vi "MultiPeak Lorentzian fit.vi"(0 "Data":cluster{dbl[], dbl[]}(graph)={[-8.499999999999992e-05, -7.999999999999991e-05, -7.500000000000001e-05, -7e-05, -6.499999999999998e-05, -5.999999999999996e-05, -5.499999999999995e-05, -4.9999999999999935e-05, -4.499999999999992e-05, -3.999999999999991e-05, -3.4999999999999895e-05, -2.999999999999999e-05, -2.4999999999999977e-05, -1.9999999999999964e-05, -1.4999999999999951e-05, -9.999999999999938e-06, -4.999999999999925e-06, 8.809142651444724e-20, 5.000000000000101e-06, 1.0000000000000114e-05, 1.5000000000000019e-05, 2.0000000000000032e-05, 2.5000000000000045e-05, 3.0000000000000167e-05, 3.499999999999996e-05, 3.9999999999999976e-05, 4.499999999999999e-05, 5e-05, 5.5000000000000016e-05, 6.000000000000003e-05, 6.500000000000003e-05, 7.000000000000005e-05, 7.500000000000006e-05, 8.000000000000007e-05, 8.500000000000009e-05, 9.00000000000001e-05, 9.500000000000011e-05, 0.00010000000000000013, 0.00010500000000000014, 0.00011000000000000015, 0.00011500000000000017, 0.00011999999999999996, 0.00012499999999999998, 0.00013, 0.000135, 0.00014000000000000001, 0.00014500000000000003, 0.00015000000000000004, 0.00015500000000000005, 0.00016000000000000007, 0.00016500000000000008, 0.0001700000000000001, 0.0001750000000000001, 0.00018000000000000012, 0.00018500000000000013, 0.00019000000000000015, 0.00019500000000000016, 0.00020000000000000017, 0.00020499999999999997, 0.00020999999999999998, 0.000215], [0.0012150575654108651, 0.001198658781387788, 0.0011426384093853204, 0.0010813452811549607, 0.0010303635282890781, 0.0009901242148328533, 0.0009655793533614787, 0.0009637788368138997, 0.0010005358746802097, 0.0010629165364520092, 0.0011453292663476753, 0.0012282965012078144, 0.0013016140805626642, 0.0013824481174704287, 0.0014643235971013074, 0.001551428490294265, 0.0016410212376952622, 0.0017011308416755618, 0.0017405751692456835, 0.0017894187526559019, 0.0018475004228560138, 0.001935889200879927, 0.0020558944722601385, 0.0022018521313563566, 0.0023273539722724924, 0.0024094326874369767, 0.0024636017852976066, 0.002504959490390853, 0.002523953570272467, 0.0025357303860099067, 0.002533784895930486, 0.002531304880465543, 0.002510967573955287, 0.0024732435245279774, 0.002443623217043697, 0.0023599211252369095, 0.0022706549323664466, 0.002214470491667274, 0.002125513838829537, 0.00201932637179927, 0.0019171339548864448, 0.0018332672503242942, 0.0017464983694980517, 0.0016410088936650942, 0.0015556613369979762, 0.0014804206312365406, 0.0014134274487672173, 0.001353115324136875, 0.001296938061612269, 0.0012362798726307397, 0.0011647776947571107, 0.0011200248904945148, 0.001093147276680698, 0.0010656806623489281, 0.0010521925231414086, 0.0010354102047782196, 0.0010134722469805815, 0.0009927942501985478, 0.0009831918813237074, 0.000993569602746048, 0.0010334011217177546]}, 1 "Enable peak doubling":bool=TRUE, 2 "range":T1={"x1"=-0.6878048780487804, "y1"=-55263.15789473684, "x 2"=0.47317073170731705, "y 2"=53947.36842105264}, 5 "Formula":string="a+4*b/(exp(1.7628*(x-c)/d)+exp(-1.7628*(x-c)/d))^2 ", 7 "Field (Oe)":dbl=39767.44186046513, 9 "model and initial parameter input\nuse \"XXX\" if void":T3={"a (constant)"="a", "b (amplitude)"="b", "c (position)"="c", "d (width)"="d", "ai"=0.0, "bi"=0.0, "ci"=0.0, "di"=0.002} {"di" format="%.3f"; "ci" format="%.3f"; "bi" format="%.3p"; "ai" format="%.2p"}, 11 "PD threshold":dbl format="%.2p", 12 "PD width":i32=10 min=3) -> (4 "Fit":cluster{dbl[], "best nonlinear fit":dbl[]}[](graph)=[{[-8.499999999999992e-05, -7.999999999999991e-05, -7.500000000000001e-05, -7e-05, -6.499999999999998e-05, -5.999999999999996e-05, -5.499999999999995e-05, -4.9999999999999935e-05, -4.499999999999992e-05, -3.999999999999991e-05, -3.4999999999999895e-05, -2.999999999999999e-05, -2.4999999999999977e-05, -1.9999999999999964e-05, -1.4999999999999951e-05, -9.999999999999938e-06, -4.999999999999925e-06, 8.809142651444724e-20, 5.000000000000101e-06, 1.0000000000000114e-05, 1.5000000000000019e-05, 2.0000000000000032e-05, 2.5000000000000045e-05, 3.0000000000000167e-05, 3.499999999999996e-05, 3.9999999999999976e-05, 4.499999999999999e-05, 5e-05, 5.5000000000000016e-05, 6.000000000000003e-05, 6.500000000000003e-05, 7.000000000000005e-05, 7.500000000000006e-05, 8.000000000000007e-05, 8.500000000000009e-05, 9.00000000000001e-05, 9.500000000000011e-05, 0.00010000000000000013, 0.00010500000000000014, 0.00011000000000000015, 0.00011500000000000017, 0.00011999999999999996, 0.00012499999999999998, 0.00013, 0.000135, 0.00014000000000000001, 0.00014500000000000003, 0.00015000000000000004, 0.00015500000000000005, 0.00016000000000000007, 0.00016500000000000008, 0.0001700000000000001, 0.0001750000000000001, 0.00018000000000000012, 0.00018500000000000013, 0.00019000000000000015, 0.00019500000000000016, 0.00020000000000000017, 0.00020499999999999997, 0.00020999999999999998, 0.000215], "best nonlinear fit"=[0.0009718951839726664, 0.0009807254858543823, 0.0009616076605343897, 0.0009333705018249478, 0.0009129931681906823, 0.000909763379760772, 0.0009260752896536717, 0.0009606338293882525, 0.0010110188438919138, 0.00107496449821926, 0.0011507542027808617, 0.0012371991520140234, 0.0013334777164069607, 0.0014389569248984503, 0.0015530359178241016, 0.0016750182813155834, 0.0018040103672834111, 0.0019388420707677372, 0.00207800877224406, 0.0022196357214930174, 0.002361468065228045, 0.0025008905889973045, 0.0026349808385329318, 0.002760597510997979, 0.0028745029297172096, 0.0029735143382420446, 0.003054674246520122, 0.003115425949217566, 0.00315377753993939, 0.0031684370891274863, 0.0031589036174095096, 0.003125503025407498, 0.0030693645891025556, 0.0029923408761758996, 0.0028968806583283737, 0.0027858693960421755, 0.002662454390667553, 0.0025298715492623517, 0.0023912882630169243, 0.002249672921582608, 0.0021076969825550677, 0.0019676711178937966, 0.001831513364386468, 0.0017007447194402514, 0.001576506285790725, 0.001459591726268164, 0.0013504891872005128, 0.0012494277072594559, 0.0011564241990958423, 0.0010713281841576634, 0.0009938624521659315, 0.0009236586396038637, 0.0008602873545952086, 0.0008032829267293593, 0.0007521631544091965, 0.0007064445906497542, 0.0006656539827412946, 0.0006293364901872711, 0.0005970612721299563, 0.000568424977978641, 0.0005430536061055539]}, {[-8.499999999999992e-05, -7.999999999999991e-05, -7.500000000000001e-05, -7e-05, -6.499999999999998e-05, -5.999999999999996e-05, -5.499999999999995e-05, -4.9999999999999935e-05, -4.499999999999992e-05, -3.999999999999991e-05, -3.4999999999999895e-05, -2.999999999999999e-05, -2.4999999999999977e-05, -1.9999999999999964e-05, -1.4999999999999951e-05, -9.999999999999938e-06, -4.999999999999925e-06, 8.809142651444724e-20, 5.000000000000101e-06, 1.0000000000000114e-05, 1.5000000000000019e-05, 2.0000000000000032e-05, 2.5000000000000045e-05, 3.0000000000000167e-05, 3.499999999999996e-05, 3.9999999999999976e-05, 4.499999999999999e-05, 5e-05, 5.5000000000000016e-05, 6.000000000000003e-05, 6.500000000000003e-05, 7.000000000000005e-05, 7.500000000000006e-05, 8.000000000000007e-05, 8.500000000000009e-05, 9.00000000000001e-05, 9.500000000000011e-05, 0.00010000000000000013, 0.00010500000000000014, 0.00011000000000000015, 0.00011500000000000017, 0.00011999999999999996, 0.00012499999999999998, 0.00013, 0.000135, 0.00014000000000000001, 0.00014500000000000003, 0.00015000000000000004, 0.00015500000000000005, 0.00016000000000000007, 0.00016500000000000008, 0.0001700000000000001, 0.0001750000000000001, 0.00018000000000000012, 0.00018500000000000013, 0.00019000000000000015, 0.00019500000000000016, 0.00020000000000000017, 0.00020499999999999997, 0.00020999999999999998, 0.000215], "best nonlinear fit"=[0.000989689814848765, 0.0009691184141790208, 0.0009366814384494319, 0.0009211036423827158, 0.0009263722031401187, 0.0009445966388776419, 0.0009696289439432098, 0.000992032437226056, 0.0010164205448619874, 0.001046657083728515, 0.0010862347078188814, 0.0011332970048991335, 0.0011997862974852938, 0.0012949918371966656, 0.001418474742517191, 0.0015812404841218492, 0.0017676702020836762, 0.001961275405311842, 0.002171201133245579, 0.0023792297464750147, 0.0025461522166526284, 0.002674004984876295, 0.0027969468914240854, 0.0029046334176933536, 0.0029750408059281484, 0.003019636865052686, 0.0030181976868652077, 0.002970402911603623, 0.0028998850653752556, 0.0028692674041395257, 0.002887874691658434, 0.0029727149791749707, 0.0030509519871012077, 0.003078767698694361, 0.00305866218326655, 0.002964500307352822, 0.0028210241662788584, 0.0026652309117736156, 0.0025033186072926125, 0.0023465893570533388, 0.002176728611772454, 0.001991535600650964, 0.0018155595228638325, 0.0016408583384044829, 0.0014856986821473453, 0.0013489469222139202, 0.0012394448202315484, 0.0011564229466427634, 0.0010753411266288153, 0.0010053852995606425, 0.0009444950046100983, 0.0008825159005678181, 0.0008246355886464278, 0.0007782164102647071, 0.0007506957685204472, 0.000728846188097151, 0.0007052979668229569, 0.000689497674504493, 0.0006869125707686534, 0.0006897761061261346, 0.0007007193940464603]}], 6 "best fit parameters":dbl[](array[numeric])=[0.00017751423776879837, 0.00038127860723276904, -8.528154856218626e-05, 3.738209460996479e-05, 0.0028135439197028837, 6.053132635732174e-05, 0.00013421483148268372], 8 "PD peak position":dbl[](array[numeric])=[-4.999999999999925e-06, 6.000000000000003e-05], 10 "# of peaks":i32=2, 14 "R-square":dbl=0.9832767875868196, 15 "std deviation":dbl[](array[numeric])=[3.738389415758166e-05, 0.00012746351087395422, 1.538590755264726e-05, 2.4846960511995104e-05, 7.093705091399118e-05, 8.710626646709724e-07, 4.935700356045006e-06])   [LabVIEW 2016]
uses:
  <vilib>/Analysis/Matrix/Datatypes/RealMatrix.ctl
  <vilib>/gmath/NumericalOptimization/Nonlinear Curve Fit LM formula string.vi
  <vilib>/gmath/NI_Gmath.lvlib
  <vilib>/Analysis/NI_AAL_SigProc.lvlib
  <vilib>/Analysis/Matrix/NI_Matrix.lvlib
panel:
  out "residue":cluster{dbl[], dbl[]}(graph)={[-8.499999999999992e-05, -7.999999999999991e-05, -7.500000000000001e-05, -7e-05, -6.499999999999998e-05, -5.999999999999996e-05, -5.499999999999995e-05, -4.9999999999999935e-05, -4.499999999999992e-05, -3.999999999999991e-05, -3.4999999999999895e-05, -2.999999999999999e-05, -2.4999999999999977e-05, -1.9999999999999964e-05, -1.4999999999999951e-05, -9.999999999999938e-06, -4.999999999999925e-06, 8.809142651444724e-20, 5.000000000000101e-06, 1.0000000000000114e-05, 1.5000000000000019e-05, 2.0000000000000032e-05, 2.5000000000000045e-05, 3.0000000000000167e-05, 3.499999999999996e-05, 3.9999999999999976e-05, 4.499999999999999e-05, 5e-05, 5.5000000000000016e-05, 6.000000000000003e-05, 6.500000000000003e-05, 7.000000000000005e-05, 7.500000000000006e-05, 8.000000000000007e-05, 8.500000000000009e-05, 9.00000000000001e-05, 9.500000000000011e-05, 0.00010000000000000013, 0.00010500000000000014, 0.00011000000000000015, 0.00011500000000000017, 0.00011999999999999996, 0.00012499999999999998, 0.00013, 0.000135, 0.00014000000000000001, 0.00014500000000000003, 0.00015000000000000004, 0.00015500000000000005, 0.00016000000000000007, 0.00016500000000000008, 0.0001700000000000001, 0.0001750000000000001, 0.00018000000000000012, 0.00018500000000000013, 0.00019000000000000015, 0.00019500000000000016, 0.00020000000000000017, 0.00020499999999999997, 0.00020999999999999998, 0.000215], [1.7794630876098662e-05, -1.1607071675361568e-05, -2.492622208495783e-05, -1.2266859442232043e-05, 1.337903494943646e-05, 3.4833259116869844e-05, 4.3553654289538125e-05, 3.13986078378035e-05, 5.401700970073583e-06, -2.830741449074488e-05, -6.451949496198033e-05, -0.00010390214711488983, -0.0001336914189216669, -0.00014396508770178466, -0.00013456117530691054, -9.377779719373417e-05, -3.634016519973491e-05, 2.2433334544104747e-05, 9.31923610015188e-05, 0.00015959402498199726, 0.00018468415142458344, 0.00017311439587899043, 0.00016196605289115363, 0.00014403590669537485, 0.00010053787621093881, 4.6122526810641554e-05, -3.647655965491412e-05, -0.00014502303761394298, -0.00025389247456413444, -0.0002991696849879606, -0.0002710289257510756, -0.0001527880462325274, -1.8412602001347846e-05, 8.642682251846145e-05, 0.00016178152493817642, 0.00017863091131064667, 0.00015856977561130555, 0.0001353593625112639, 0.0001120303442756882, 9.691643547073093e-05, 6.903162921738631e-05, 2.3864482757167318e-05, -1.5953841522635404e-05, -5.988638103576857e-05, -9.080760364337968e-05, -0.00011064480405424378, -0.00011104436696896436, -9.30047606166925e-05, -8.108307246702698e-05, -6.594288459702089e-05, -4.9367447555833245e-05, -4.1142739036045665e-05, -3.565176594878079e-05, -2.5066516464652207e-05, -1.4673858887493448e-06, 2.2401597447396803e-05, 3.964398408166231e-05, 6.016118431722195e-05, 8.985129863869705e-05, 0.0001213511281474936, 0.0001576657879409064]}
  out "covariance":T2=[[0.09601636295019793, -0.11196924282221532, 0.0019290808585169803, -0.008016159684207873, -0.15830836798965434, -0.0003679452768878755, -0.01111098483349951], [-0.11196924282221542, 1.1162151876482052, -0.09483397785102357, 0.10825444863719698, 0.20981268047054838, 0.0013201880795881457, 0.009063931764684398], [0.001929080858517002, -0.09483397785102358, 0.01626381447167083, -0.023123770063261814, -0.005876578599017109, -0.00015274264582045002, 0.000286765518797958], [-0.008016159684207928, 0.10825444863719715, -0.023123770063261818, 0.042415316674133494, 0.02100058943438996, 0.0003972550480277107, -0.00044102254426060404], [-0.15830836798965442, 0.20981268047054832, -0.005876578599017081, 0.021000589434389854, 0.34571835125452366, 0.0007469589653986517, 0.014676057612944117], [-0.0003679452768878726, 0.0013201880795881745, -0.00015274264582044948, 0.00039725504802770573, 0.0007469589653986541, 5.212846938596066e-05, 2.0363029410124748e-05], [-0.0111109848334995, 0.009063931764684367, 0.0002867655187979612, -0.00044102254426061195, 0.014676057612944087, 2.0363029410124728e-05, 0.0016736850862781277]] format="%#_5g"
  out "Initial parameters":dbl[](array[numeric])=[0.0, 0.0016410212376952622, -4.999999999999925e-06, 0.002, 0.0025357303860099067, 6.000000000000003e-05, 0.002]
  out "PD Amplitudes":dbl[](array[numeric])=[0.0016410212376952622, 0.0025357303860099067]
  in  "model description output":T4={"model"="a+4*b0/(exp(1.7628*(x-c0)/d0)+exp(-1.7628*(x-c0)/d0))^2 +a+4*b1/(exp(1.7628*(x-c1)/d1)+exp(-1.7628*(x-c1)/d1))^2 ", "Parameters"=["a", "b0", "c0", "d0", "b1", "c1", "d1"], "x"="x"}
  # "This program can fit any peak function as far as the number of parameters<=4\nuse \"XXX\" and \"NaN\" if the corresponding parameter is not in use.\n\n4 parameter functions:\nLorentzian: a+b*d^2/(4*x^2-8*c*x+4*c^2+d^2)\n\nHyperbolic cosine: a+4*b/(exp(1.7628*(x-c)/d)+exp(-1.7628*(x-c)/d))^2"
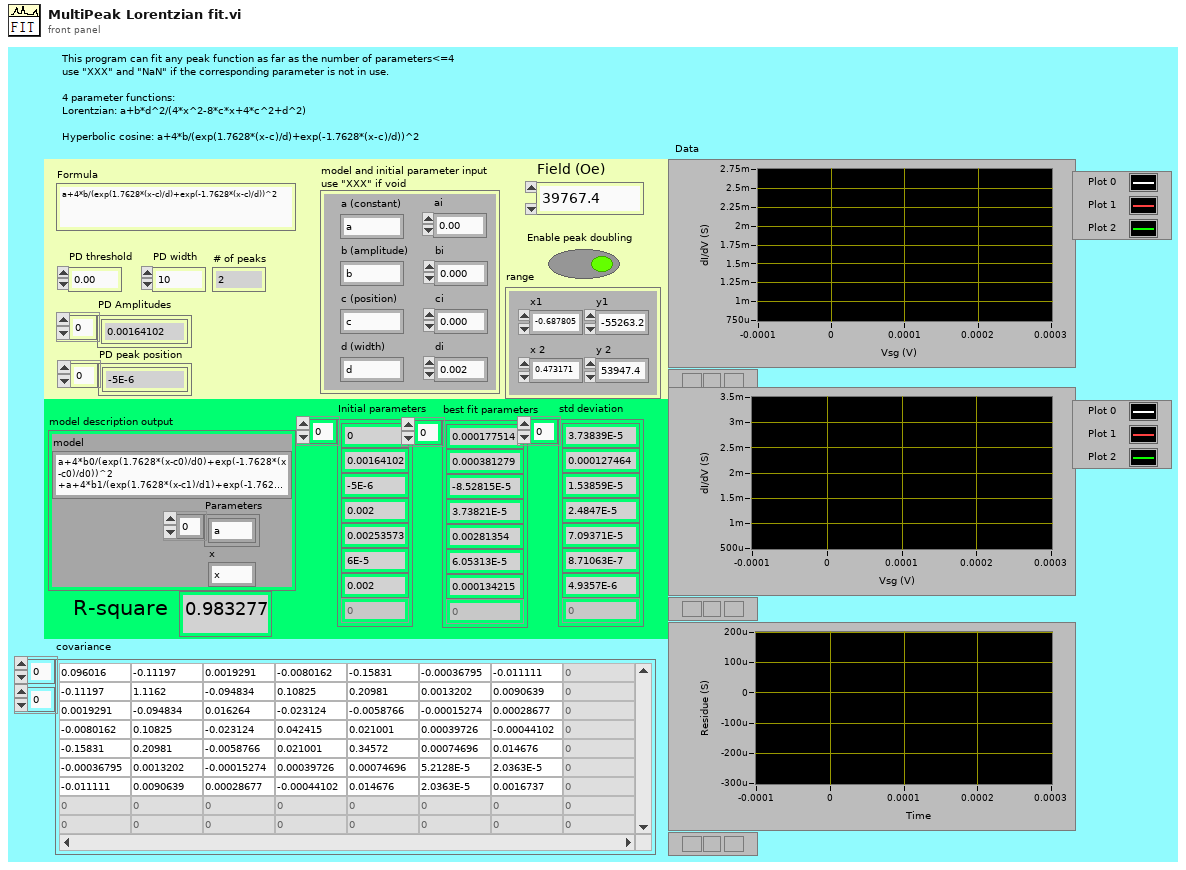
[diagram p1: front panel]
types:
  T1 = cluster{"x1":dbl, "y1":dbl, "x 2":dbl, "y 2":dbl}
  T2 = typedef "NI_Matrix.lvlib/RealMatrix.ctl" = dbl[][]
  T3 = cluster{"a (constant)":string, "b (amplitude)":string, "c (position)":string, "d (width)":string, "ai":dbl, "bi":dbl, "ci":dbl, "di":dbl}
  T4 = cluster{"model":string, "Parameters":string[], "x":string}
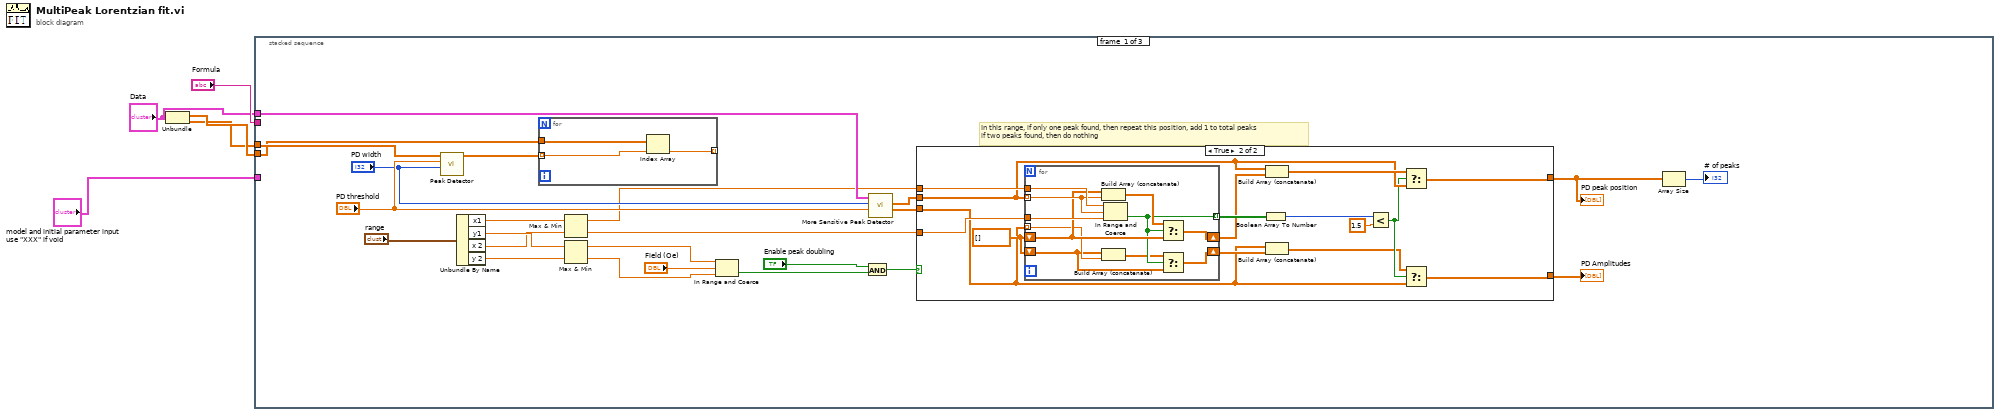
[diagram p0: block diagram]
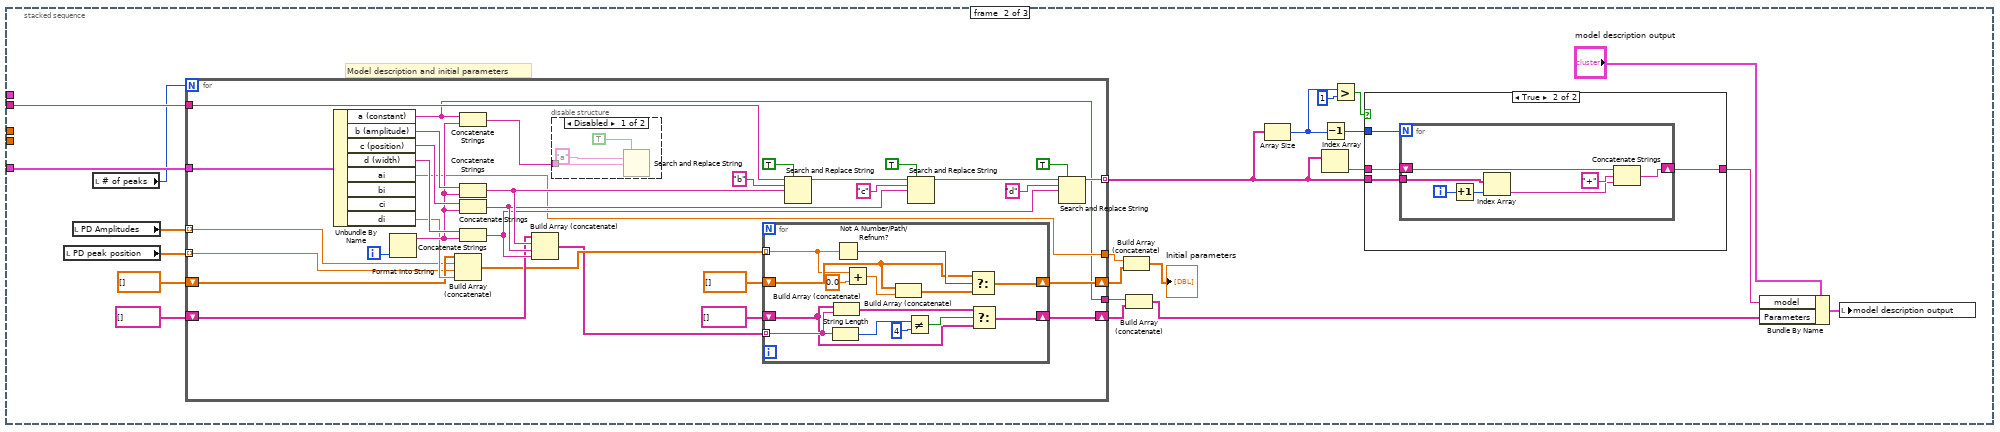
[diagram p3: hidden frame]
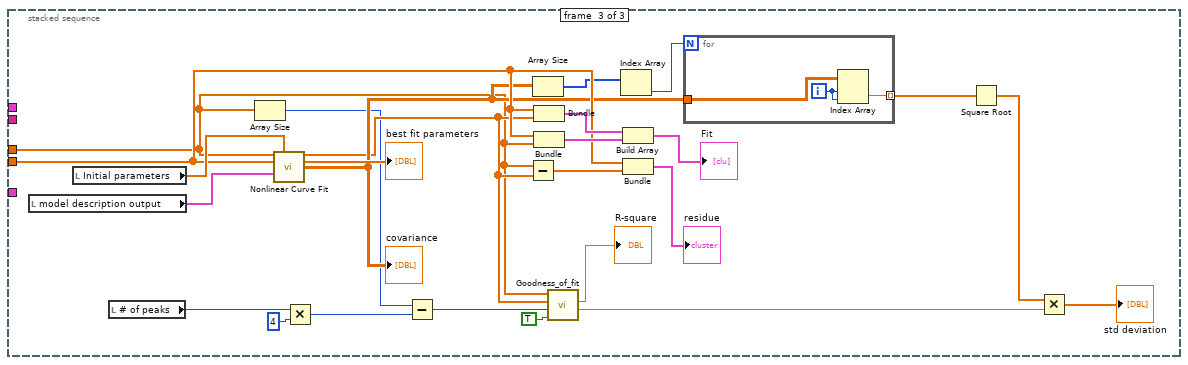
[diagram p6: hidden frame]
diagram:
  n1 = Unbundle("Data") -> (w3:dbl[], w1:dbl[])
  n2 = stacked-sequence {
    tunnel: "Formula" -> [_ w82 _]
    tunnel: "model and initial parameter input\nuse \"XXX\" if void" -> [_ w81 _]
    tunnel: w3 -> [w27 _ w162]
    tunnel: w1 -> [w29 _ w154]
    tunnel: "Data" -> [w25 _ _]
    frame #0 {
      # "In this range, if only one peak found, then repeat this position, add 1 to total peaks\nif two peaks found, then do nothing"
      n3 = call <vilib>:"Peak Detector.vi"("width"="PD width", "threshold"="PD threshold", "X"=w29) -> ("Locations"=w26:dbl[])  [unwired: 4 in, 4 out]
      n4 = Unbundle By Name("range") -> ("x1"=w9:dbl, "y1"=w16:dbl, "x 2"=w8:dbl, "y 2"=w15:dbl)
      n5 = for {
        tunnel: w27 -> [w60]
        tunnel: w26 -> [w59] mode=indexing
        tunnel: [w58] -> _ mode=indexing
        n6 = Index Array(array=w60, index=w59) -> (element=w58:dbl)
      }
      n7 = Max & Min(x=w9, y=w8) -> (max(x,y)=w7:dbl, min(x,y)=w6:dbl)
      n8 = Max & Min(x=w16, y=w15) -> (max(x,y)=w14:dbl, min(x,y)=w13:dbl)
      n9 = In Range and Coerce(upper limit=w14, x="Field (Oe)", lower limit=w13) -> (In Range?=w11:bool)  [unwired: 1 out]
      n10 = And(x="Enable peak doubling", y=w11) -> (x .and. y?=w10:bool)
      n11 = call "More Sensitive Peak Detector.vi"("PD threshold"="PD threshold", "Smooth points"="PD width", "Input XY"=w25) -> ("Amplitudes"=w19:dbl[], "Positions"=w21:dbl[])  [unwired: 6 in, 1 out]
      n12 = case shown="True" w10 {
        tunnel: w21 -> [w31 w37]
        tunnel: [w31 w36] -> w20
        tunnel: w19 -> [w30 w32]
        tunnel: [w30 w33] -> w18
        tunnel: w7 -> [_ w46]
        tunnel: w6 -> [_ w45]
        frame False {
        }
        frame True {
          w40 = dbl[] []
          n13 = for {
            tunnel: w37 -> [w55] mode=indexing
            shift-right: [w53] -> w41
            shift-left: w40 -> [w52]
            tunnel: w46 -> [w57]
            tunnel: w45 -> [w56]
            tunnel: [w51] -> w44 mode=indexing
            shift-right: [w48] -> w39
            shift-left: w40 -> [w47]
            tunnel: w32 -> [w50] mode=indexing
            n14 = Build Array (concatenate)(w52, w55) -> (w54:dbl[])
            n15 = Build Array (concatenate)(w47, w50) -> (w49:dbl[])
            n16 = In Range and Coerce(upper limit=w57, x=w55, lower limit=w56) -> (In Range?=w51:bool)  [unwired: 1 out]
            n17 = Select(t=w54, s=w51, f=w52) -> (s? t:f=w53:dbl[])
            n18 = Select(t=w49, s=w51, f=w47) -> (s? t:f=w48:dbl[])
          }
          n19 = Boolean Array To Number(Boolean array=w44) -> (number=w43:u32)
          n20 = Build Array (concatenate)(w37, w41) -> (w38:dbl[])
          n21 = Build Array (concatenate)(w32, w39) -> (w34:dbl[])
          n22 = Less?(x=w43, y=1.5) -> (x < y?=w35:bool)
          n23 = Select(t=w38, s=w35, f=w37) -> (s? t:f=w36:dbl[])
          n24 = Select(t=w34, s=w35, f=w32) -> (s? t:f=w33:dbl[])
        }
      }
      "PD Amplitudes" <- w18
      "PD peak position" <- w20
      n25 = Array Size(array=w20) -> (size(s)=→"# of peaks":i32)
    }
    frame #1 {
      # "Model description and initial parameters"
      n26 = local read "PD peak position"() -> (w68:dbl[])
      n27 = local read "PD Amplitudes"() -> (w67:dbl[])
      n28 = local read "# of peaks"() -> (w70:i32)
      n29 = for {
        N: w70 -> [_]
        tunnel: w82 -> [w97]
        tunnel: w81 -> [w127]
        tunnel: [w113] -> w76 mode=indexing
        shift-right: [w98] -> w62
        shift-left: string[] [] -> [w108]
        shift-right: [w101] -> w65
        shift-left: dbl[] [] -> [w106]
        tunnel: w68 -> [w105] mode=indexing
        tunnel: w67 -> [w104] mode=indexing
        tunnel: [w96] -> w66
        tunnel: [w95] -> w63
        i -> [w126]
        n30 = Unbundle By Name(w127) -> ("a (constant)"=w95:string, "b (amplitude)"=w125:string, "c (position)"=w124:string, "d (width)"=w123:string, "ai"=w96:dbl, "di"=w107:dbl)  [unwired: 2 out]
        n31 = Format Into String(w126) -> (resulting string=w122:string)  [unwired: 3 in, 1 out]
        n32 = Build Array (concatenate)(w106, w104, w105, w107) -> (w103:dbl[])
        n33 = Concatenate Strings(w95, w122) -> (w112:string)
        n34 = Concatenate Strings(w125, w122) -> (w111:string)
        n35 = Concatenate Strings(w124, w122) -> (w110:string)
        n36 = Concatenate Strings(w123, w122) -> (w109:string)
        n37 = Build Array (concatenate)(w108, w111, w110, w109) -> (w100:string[])
        n38 = disable-structure shown="Disabled" {
          disable-tunnel: w112 -> [w128 _]
          frame Disabled {
            n39 = Search and Replace String(replace all?=TRUE ("replace all? (F)"), search string="a" ("substring (\"\")"), replace string=w128) -> ()  [unwired: 5 in, 4 out]
          }
          frame Enabled {
          }
        }
        n40 = for {
          tunnel: w103 -> [w133] mode=indexing
          shift-right: [w143] -> w101
          shift-left: dbl[] [] -> [w142]
          tunnel: w100 -> [w137] mode=indexing
          shift-right: [w134] -> w98
          shift-left: string[] [] -> [w135]
          n41 = String Length(string=w137) -> (length=w140:i32)
          n42 = Build Array (concatenate)(w135, w137) -> (w136:string[])
          n43 = Not A Number/Path/Refnum?(number/path/refnum=w133) -> (NaN/Path/Refnum?=w144:bool)
          n44 = Add(x=w133, y=0.0) -> (x+y=w131:dbl)
          n45 = Build Array (concatenate)(w142, w131) -> (w141:dbl[])
          n46 = Not Equal?(x=w140, y=4) -> (x != y?=w138:bool)
          n47 = Select(t=w142, s=w144, f=w141) -> (s? t:f=w143:dbl[])
          n48 = Select(t=w136, s=w138, f=w135) -> (s? t:f=w134:string[])
        }
        n49 = Search and Replace String(replace all?=TRUE ("replace all? (F)"), input string=w97, search string="b", replace string=w111) -> (result string=w118:string)  [unwired: 4 in, 3 out]
        n50 = Search and Replace String(replace all?=TRUE ("replace all? (F)"), input string=w118, search string="c", replace string=w110) -> (result string=w117:string)  [unwired: 4 in, 3 out]
        n51 = Search and Replace String(replace all?=TRUE ("replace all? (F)"), input string=w117, search string="d", replace string=w109) -> (result string=w113:string)  [unwired: 4 in, 3 out]
      }
      n52 = Build Array (concatenate)(w66, w65) -> (→"Initial parameters":dbl[])
      n53 = Build Array (concatenate)(w63, w62) -> (w61:string[])
      n54 = Array Size(array=w76) -> (size(s)=w78:i32)
      n55 = Decrement(x=w78) -> (x-1=w77:i32)
      n56 = Index Array(array=w76) -> (element=w75:string)  [unwired: 1 in]
      n57 = Greater?(x=w78, y=1) -> (0:w79:bool)
      n58 = case shown="True" w79 {
        tunnel: w76 -> [_ w87]
        tunnel: w77 -> [_ w86]
        tunnel: w75 -> [w83 w85]
        tunnel: [w83 w84] -> w73
        frame False {
        }
        frame True {
          n59 = for {
            N: w86 -> [_]
            tunnel: w87 -> [w91]
            shift-right: [w88] -> w84
            shift-left: w85 -> [w93]
            i -> [w94]
            n60 = Increment(x=w94) -> (x+1=w92:i32)
            n61 = Index Array(array=w91, index=w92) -> (element=w89:string)
            n62 = Concatenate Strings(w93, "+" ("string"), w89) -> (w88:string)
          }
        }
      }
      n63 = Bundle By Name(cluster="model description output", "model"=w73, "Parameters"=w61) -> (w72:T4)
      n64 = local write "model description output"(w72) -> ()
    }
    frame #2 {
      n65 = local read "model description output"() -> (w169:T4)
      n66 = local read "Initial parameters"() -> (w168:dbl[])
      n67 = local read "# of peaks"() -> (w153:i32)
      n68 = Array Size(array=w154) -> (size(s)=w147:i32)
      n69 = call-poly <vilib>:"Nonlinear Curve Fit.vi"("Y"=w154, "initial parameters"=w168, "X"=w162, "model description"=w169) -> ("best nonlinear fit"=w155:dbl[], "best fit parameters"=→"best fit parameters":dbl[], "covariance"=w156:T2)  [unwired: 7 in, 2 out]
      "covariance" <- w156
      n70 = Multiply(x=w153, y=4) -> (x*y=w151:i32)
      n71 = Subtract(x=w147, y=w151) -> (x-y=w146:i32)
      n72 = Subtract(x=w154, y=w155) -> (x-y=w163:dbl[])
      n73 = Array Size(array=w156) -> (size(s)=w160:i32[])
      n74 = Bundle(w162, "best nonlinear fit"=w155) -> (w164:cluster{dbl[], "best nonlinear fit":dbl[]})  [unwired: 1 in]
      n75 = Bundle(w162, w154) -> (w165:cluster{dbl[], dbl[]})  [unwired: 1 in]
      n76 = call "Goodness_of_fit.vi"("Wight=1"=TRUE, "degree of freedom"=w146, "Best Fit"=w155, "Y"=w154) -> ("RMSE"=w149:dbl, "R-square"=→"R-square":dbl)  [unwired: 5 in, 1 out]
      n77 = Index Array(array=w160) -> (element=w159:i32)  [unwired: 1 in]
      n78 = Build Array(w164, w165) -> (→"Fit":cluster{dbl[], "best nonlinear fit":dbl[]}[])
      n79 = Bundle(w162, w163) -> (→"residue":cluster{dbl[], dbl[]})  [unwired: 1 in]
      n80 = for {
        N: w159 -> [_]
        tunnel: w156 -> [w172]
        tunnel: [w170] -> w158 mode=indexing
        i -> [w171]
        n81 = Index Array(array=w172, index (row)=w171, index (col)=w171) -> (element=w170:dbl)
      }
      n82 = Square Root(x=w158) -> (sqrt(x)=w157:dbl[])
      n83 = Multiply(x=w157, y=w149) -> (x*y=→"std deviation":dbl[])
    }
  }
